vi "set_enabled_state.vi"(8 "error in (no error)":errorcluster, 10 "enabled?":bool, 11 "GenericClock in":refnum<class "GenericClock.lvclass">) -> (0 "error out":errorcluster, 3 "GenericClock out":refnum<class "GenericClock.lvclass">)   [LabVIEW 2017, in "GenericClock.lvclass"]
uses:
  GenericClock.lvclass
  GenericClock.lvclass/GenericClock.ctl
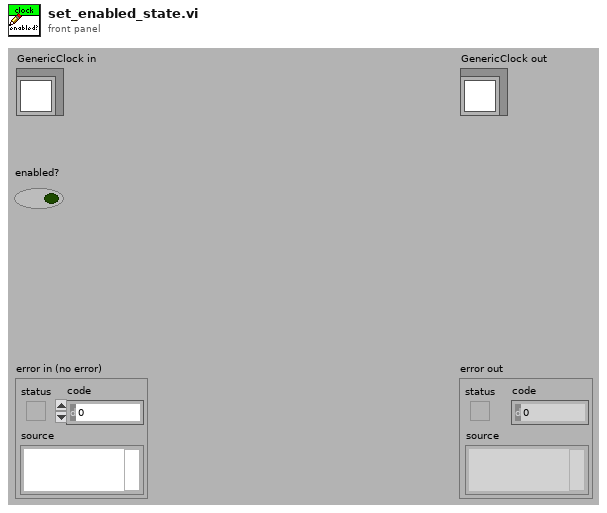
[diagram p1: front panel]
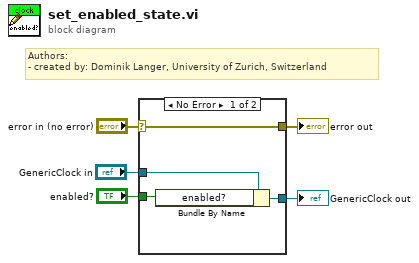
[diagram p0: block diagram]
diagram:
  # "Authors: \n- created by: Dominik Langer, University of Zurich, Switzerland"
  n1 = case shown="No Error" "error in (no error)" {
    selector: "error in (no error)" -> [w9 w11]
    tunnel: [w9 w11] -> w4
    tunnel: [w6 w10] -> w2
    tunnel: "GenericClock in" -> [w7 w10]
    tunnel: "enabled?" -> [w8 _]
    frame No Error {
      n2 = Bundle By Name(cluster=w7, "enabled?"=w8) -> (w6:refnum<class "GenericClock.lvclass">)
    }
    frame Error {
    }
  }
  "error out" <- w4
  "GenericClock out" <- w2
